vi "PQconnectStart.vi"(8 "error in (no error)":errorcluster, 11 "conninfo":string) -> (0 "error out":errorcluster, 3 "return type":u32)   [LabVIEW 2019, in "libpqlv.lvlib"]
uses:
  libpqlv.lvlib
  libpq.dll
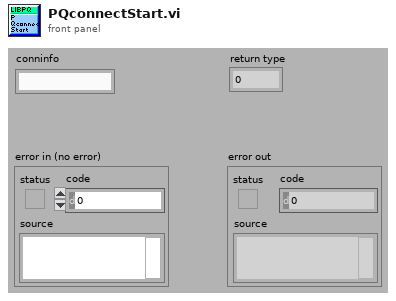
[diagram p1: front panel]
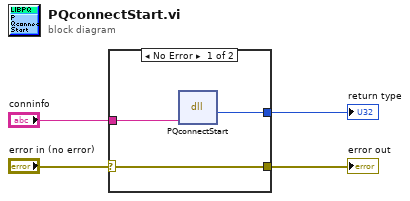
[diagram p0: block diagram]
diagram:
  n1 = case shown="No Error" "error in (no error)" {
    selector: "error in (no error)" -> [w7 w8]
    tunnel: [w7 w8] -> w3
    tunnel: [w6 _] -> w2
    tunnel: "conninfo" -> [w5 _]
    frame No Error {
      n2 = dll-call lib="libpq.*" fn="PQconnectStart"("conninfo"=w5) -> ("return type"=w6:u32)  [unwired: 4 in, 2 out]
    }
    frame Error {
    }
  }
  "return type" <- w2
  "error out" <- w3
